vi "Xml_Load_Sequence.vi"(7 "Version String":string, 8 "error in (no error)":errorcluster, 10 "XML Path":path=path "D:/TEST.xml", 11 "Refnum Clust":refnum<vi>) -> (0 "error out":errorcluster)   [LabVIEW 2018]
uses:
  controls/SEQUENCE_Inputs.ctl
  controls/EXCIT_Inputs.ctl
  controls/DATA_Inputs.ctl
  controls/TIMING_Inputs.ctl
  controls/PROCESSING_Inputs.ctl
  controls/TRAPPING_Inputs.ctl
panel:
  in  "SEQUENCE Inputs":T1={"EXCIT Inputs"={"Number of Excitations"=1, "Script Text"="", "Table of Waveforms"=[]}, "DATA Inputs"={"Record Length"=524000, "Sample Rate"=2000000.0, "Data Type"=0, "Vertical Range"=10.0, "Acquisition Duration"=262.0}, "TIMING Inputs"={"Number of Acquisitions "=1, "Number of Accumulations"=1, "Table of Waveforms"=[], "Script Text"=""}, "PROCESSING Inputs"={"Reference Mass"=300.0939, "Cyclotron Freq"=255.727, "Magnetron Freq"=0.001}, "TRAPPING Inputs"={"Number of Channels"=4, "Init Values"=[2.0, 9.0, 2.0, 9.0], "Opening Values"=[0.0, 0.0, 0.0, 0.0], "Trapping Values"=[2.0, 9.0, 2.0, 9.0], "Emptying Values"=[-10.0, -10.0, -10.0, -10.0], "Adiabatic ON"=FALSE, "Adiabatic Duration"=100, "Adiabatic Waveforms"=["Adiabatic_None_2_2_2000", "Adiabatic_Ramp_9_0_2000", "Adiabatic_None_2_2_2000", "Adiabatic_RC_9_0_2000"], "Ions Refill ON"=FALSE, "Number of Ions Refills"=1, "Trapping Delay"=400.0, "Trapping Duration"=300.0}} {"TRAPPING Inputs"."Trapping Duration" min=2.0; "TRAPPING Inputs"."Trapping Delay" min=2.0; "TRAPPING Inputs"."Number of Ions Refills" min=1 max=1000; "TRAPPING Inputs"."Trapping Values" min=-10.0 max=10.0; "TRAPPING Inputs"."Init Values" min=-10.0 max=10.0; "TRAPPING Inputs"."Emptying Values" min=-10.0 max=10.0; "TRAPPING Inputs"."Opening Values" min=-10.0 max=10.0; "PROCESSING Inputs"."Magnetron Freq" format="%.5g"; "PROCESSING Inputs"."Cyclotron Freq" format="%.5g"; "PROCESSING Inputs"."Reference Mass" format="%.5g"; "TIMING Inputs"."Number of Accumulations" min=0 max=50 step=1; "TIMING Inputs"."Number of Acquisitions" min=1 max=10 step=1; "DATA Inputs"."Vertical Range" items=["0.2"=0.2, "0.4"=0.4, "1"=1.0, "2"=2.0, "4"=4.0, "10"=10.0]; "DATA Inputs"."Data Type" items=["I16", "DBL"]; "DATA Inputs"."Sample Rate" items=["1 MHz"=1000000.0, "2 MHz"=2000000.0, "5 MHz"=5000000.0, "10 MHz"=10000000.0, "20 MHz"=20000000.0, "25 MHz"=25000000.0, "50 MHz"=50000000.0, "100 MHz"=100000000.0]; "EXCIT Inputs"."Number of Excitations" min=1 max=10}
  # "GO_out"
  # "Gout"
  # "GI_in"
  # "Gin"
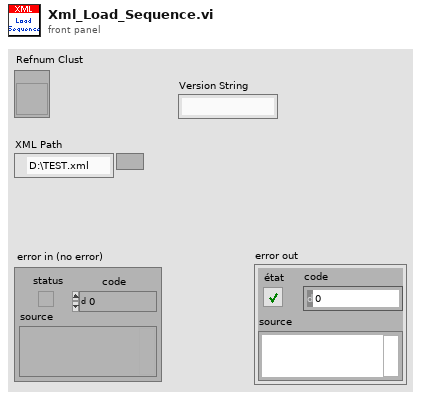
[diagram p1: front panel]
types:
  T1 = typedef "SEQUENCE_Inputs.ctl" = cluster{"EXCIT Inputs":T2, "DATA Inputs":T3, "TIMING Inputs":T4, "PROCESSING Inputs":T5, "TRAPPING Inputs":T6}
  T2 = typedef "EXCIT_Inputs.ctl" = cluster{"Number of Excitations":i32, "Script Text":string, "Table of Waveforms":string[]}
  T3 = typedef "DATA_Inputs.ctl" = cluster{"Record Length":i32, "Sample Rate":dbl, "Data Type":u8, "Vertical Range":dbl, "Acquisition Duration":dbl}
  T4 = typedef "TIMING_Inputs.ctl" = cluster{"Number of Acquisitions ":i16, "Number of Accumulations":i16, "Table of Waveforms":string[], "Script Text":string}
  T5 = typedef "PROCESSING_Inputs.ctl" = cluster{"Reference Mass":dbl, "Cyclotron Freq":dbl, "Magnetron Freq":dbl}
  T6 = typedef "TRAPPING_Inputs.ctl" = cluster{"Number of Channels":i32, "Init Values":dbl[], "Opening Values":dbl[], "Trapping Values":dbl[], "Emptying Values":dbl[], "Adiabatic ON":bool, "Adiabatic Duration":i32, "Adiabatic Waveforms":string[], "Ions Refill ON":bool, "Number of Ions Refills":i32, "Trapping Delay":dbl, "Trapping Duration":dbl}
  T7 = cluster{"Number of Channels":i32, "Init Values":dbl[], "Opening Values":dbl[], "Trapping Values":dbl[], "Emptying Values":dbl[], "Adiabatic ON":bool, "Adiabatic Duration":i32, "Adiabatic Waveforms":string[]}
  T8 = cluster{"Number Of Acquisitions ":i16, "Number Of Accumulations":i16, "Number Of Loops":i16, "Table of Waveforms":string[], "Script text":string}
  T9 = cluster{"Record Length":i32, "Sample Rate":dbl, "Type Of Data":u8, "Vertical Range":dbl, "Acquisition Duration":dbl}
  T10 = cluster{"Number of Excitations":i32, "Script text":string, "Table of Waveforms":string[]}
  T11 = cluster{"Reference Mass":dbl, "Cyclotron Freq":dbl, "Magnetron Freq":dbl}
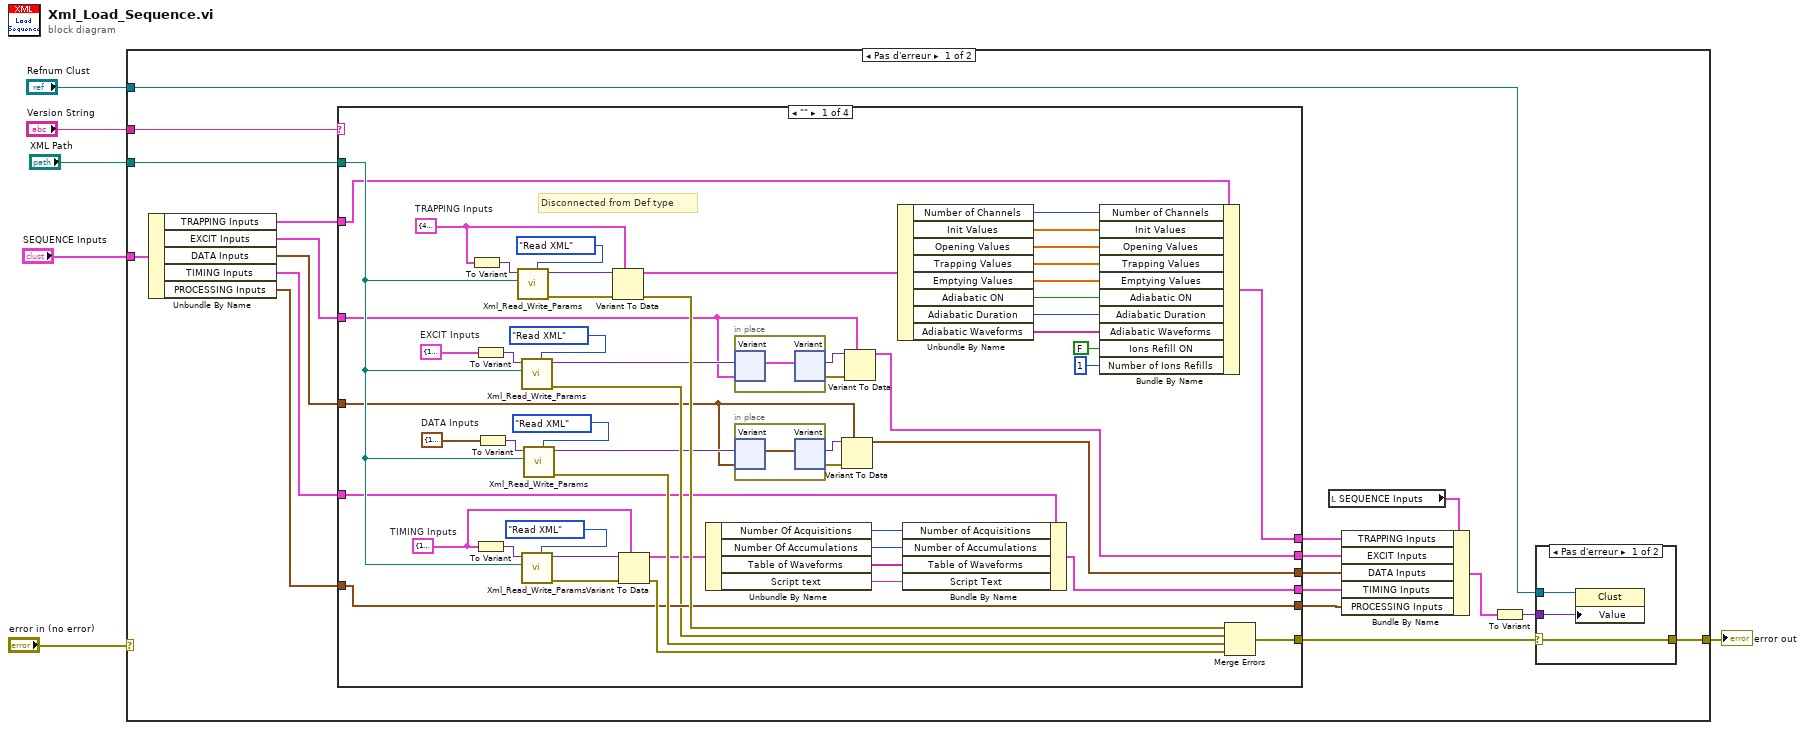
[diagram p0: block diagram]
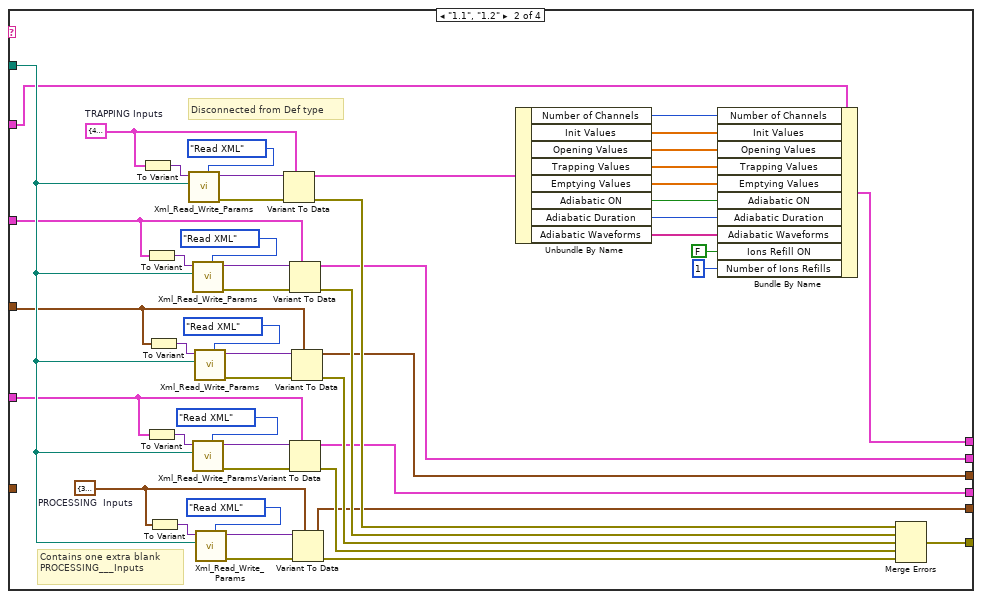
[diagram p2: hidden frame]
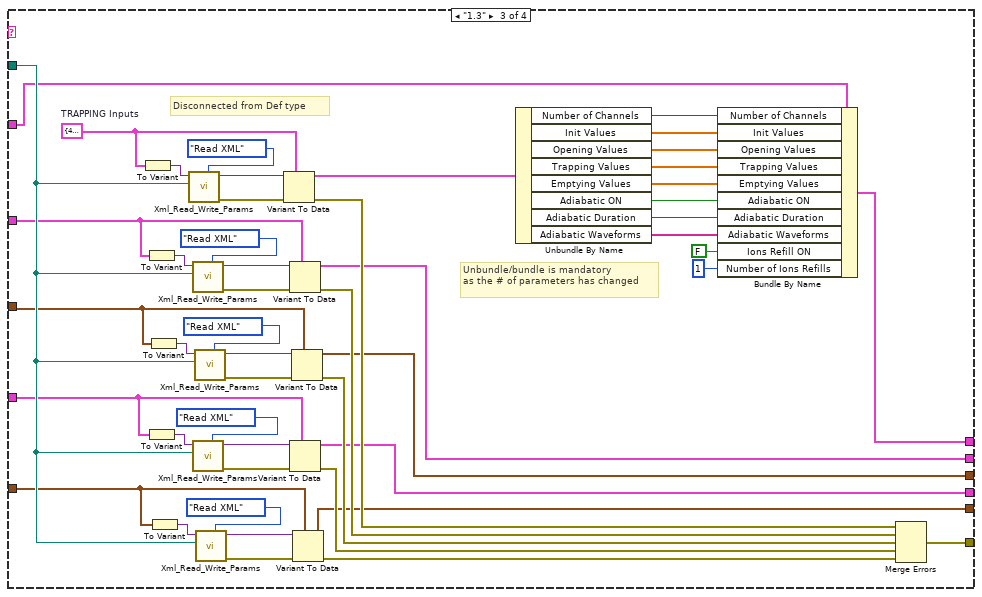
[diagram p3: hidden frame]
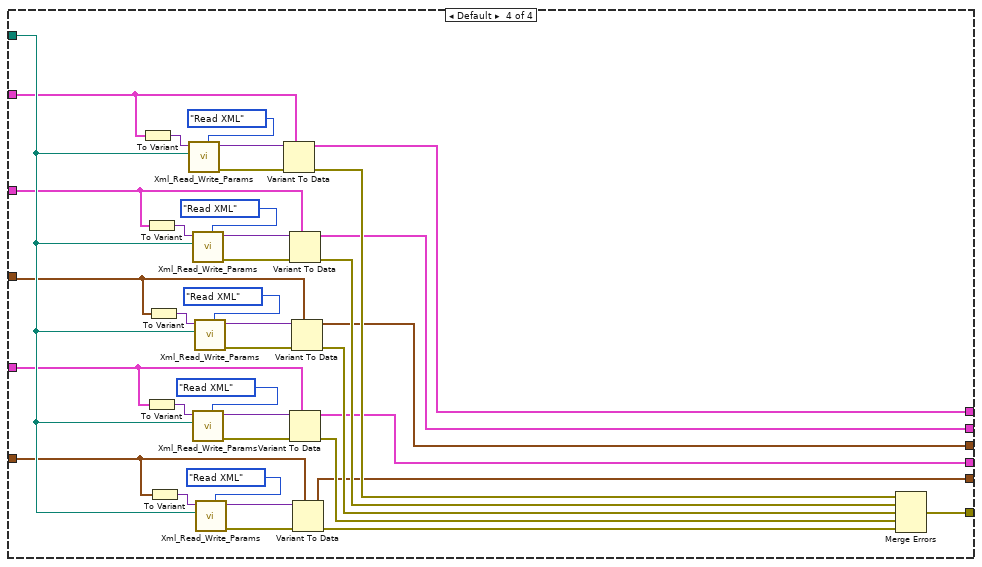
[diagram p4: hidden frame]
diagram:
  n1 = case shown="Pas d'erreur" "error in (no error)" {
    selector: "error in (no error)" -> [_ w220]
    tunnel: "XML Path" -> [w25 _]
    tunnel: [w22 w220] -> w4
    tunnel: "Version String" -> [w24 _]
    tunnel: "Refnum Clust" -> [w21 _]
    tunnel: "SEQUENCE Inputs" -> [w20 _]
    frame No Error {
      n2 = Unbundle By Name(w20) -> ("TRAPPING Inputs"=w19:T6, "EXCIT Inputs"=w18:T2, "DATA Inputs"=w17:T3, "TIMING Inputs"=w16:T4, "PROCESSING Inputs"=w15:T5)
      n3 = case shown="\"\"" w24 {
        tunnel: w25 -> [w62 w104 w153 w190]
        tunnel: [w78 w129 w178 w215] -> w23
        tunnel: w19 -> [w59 w92 w131 w188]
        tunnel: w18 -> [w52 w102 w151 w187]
        tunnel: w17 -> [w46 w101 w150 w186]
        tunnel: w16 -> [w39 w100 w149 w185]
        tunnel: w15 -> [w58 _ w148 w184]
        tunnel: [w60 w93 w133 w183] -> w14
        tunnel: [w37 w99 w147 w182] -> w9
        tunnel: [w47 w98 w146 w181] -> w8
        tunnel: [w38 w97 w145 w180] -> w13
        tunnel: [w58 w96 w144 w179] -> w12
        frame "" {
          w36 = T7 {"Number of Channels"=4, "Init Values"=[2.0, 9.0, 2.0, 9.0], "Opening Values"=[0.0, 0.0, 0.0, 0.0], "Trapping Values"=[2.0, 9.0, 2.0, 9.0], "Emptying Values"=[-10.0, -10.0, -10.0, -10.0], "Adiabatic ON"=FALSE, "Adiabatic Duration"=100, "Adiabatic Waveforms"=["Adiabatic_None_2_2_2000", "Adiabatic_Ramp_9_0_2000", "Adiabatic_None_2_2_2000", "Adiabatic_RC_9_0_2000"]}  # TRAPPING Inputs
          w45 = T8 {"Number Of Acquisitions "=1, "Number Of Accumulations"=1, "Number Of Loops"=1, "Table of Waveforms"=[], "Script text"=""}  # TIMING Inputs
          w51 = T9 {"Record Length"=100000, "Sample Rate"=10000000.0, "Type Of Data"=0, "Vertical Range"=10.0, "Acquisition Duration"=100000.0}  # DATA Inputs
          w57 = T10 {"Number of Excitations"=1, "Script text"="", "Table of Waveforms"=[]}  # EXCIT Inputs
          # "Disconnected from Def type"
          n4 = To Variant(anything=w36) -> (Variant=w77:variant)
          n5 = To Variant(anything=w57) -> (Variant=w72:variant)
          n6 = To Variant(anything=w45) -> (Variant=w65:variant)
          n7 = To Variant(anything=w51) -> (Variant=w71:variant)
          n8 = call "Xml_Read_Write_Params.vi"("Variant"=w77, "XML Path"=w62, "Command"=enum16{"Read XML", "Set", "Get", "Write XML"}."Read XML") -> ("Variant Output"=w75:variant, "error out"=w76:errorcluster)  [unwired: 4 in, 1 out]
          n9 = call "Xml_Read_Write_Params.vi"("Variant"=w72, "XML Path"=w62, "Command"=enum16{"Read XML", "Set", "Get", "Write XML"}."Read XML") -> ("Variant Output"=w55:variant, "error out"=w56:errorcluster)  [unwired: 4 in, 1 out]
          n10 = call "Xml_Read_Write_Params.vi"("Variant"=w65, "XML Path"=w62, "Command"=enum16{"Read XML", "Set", "Get", "Write XML"}."Read XML") -> ("Variant Output"=w67:variant, "error out"=w66:errorcluster)  [unwired: 4 in, 1 out]
          n11 = call "Xml_Read_Write_Params.vi"("Variant"=w71, "XML Path"=w62, "Command"=enum16{"Read XML", "Set", "Get", "Write XML"}."Read XML") -> ("Variant Output"=w50:variant, "error out"=w70:errorcluster)  [unwired: 4 in, 1 out]
          n12 = Variant To Data(error in=w76, type=w36, Variant=w75) -> (data=w35:T7, error out=w63:errorcluster)
          n13 = Variant To Data(error in=w66, type=w45, Variant=w67) -> (data=w40:T8, error out=w64:errorcluster)
          n14 = Unbundle By Name(w40) -> ("Number Of Acquisitions"=w44:i16, "Number Of Accumulations"=w43:i16, "Table of Waveforms"=w42:string[], "Script text"=w41:string)
          n15 = in-place "Structure Élément en place" {
            n16 = in-place-variant #1(w55, w52) -> (w80:T2)  [unwired: 1 out]
            n17 = in-place-variant #1(w80) -> (w53:variant, w54:errorcluster)
          }
          n18 = in-place "Structure Élément en place" {
            n19 = in-place-variant #2(w50, w46) -> (w79:T3)  [unwired: 1 out]
            n20 = in-place-variant #2(w79) -> (w48:variant, w49:errorcluster)
          }
          n21 = Variant To Data(error in=w49, type=w46, Variant=w48) -> (data=w47:T3)  [unwired: 1 out]
          n22 = Variant To Data(error in=w54, type=w52, Variant=w53) -> (data=w37:T2)  [unwired: 1 out]
          n23 = Unbundle By Name(w35) -> ("Number of Channels"=w34:i32, "Init Values"=w33:dbl[], "Opening Values"=w32:dbl[], "Trapping Values"=w31:dbl[], "Emptying Values"=w30:dbl[], "Adiabatic ON"=w29:bool, "Adiabatic Duration"=w28:i32, "Adiabatic Waveforms"=w27:string[])
          n24 = Bundle By Name(cluster=w39, "Number of Acquisitions"=w44, "Number of Accumulations"=w43, "Table of Waveforms"=w42, "Script Text"=w41) -> (w38:T4)
          n25 = Bundle By Name(cluster=w59, "Number of Channels"=w34, "Init Values"=w33, "Opening Values"=w32, "Trapping Values"=w31, "Emptying Values"=w30, "Adiabatic ON"=w29, "Adiabatic Duration"=w28, "Adiabatic Waveforms"=w27, "Ions Refill ON"=FALSE ("Ions Accumulation ON"), "Number of Ions Refills"=1) -> (w60:T6)
          n26 = Merge Errors(w63, w56, w70, w64) -> (w78:errorcluster)
        }
        frame "1.1", "1.2" {
          w90 = T7 {"Number of Channels"=4, "Init Values"=[2.0, 9.0, 2.0, 9.0], "Opening Values"=[0.0, 0.0, 0.0, 0.0], "Trapping Values"=[2.0, 9.0, 2.0, 9.0], "Emptying Values"=[-10.0, -10.0, -10.0, -10.0], "Adiabatic ON"=FALSE, "Adiabatic Duration"=100, "Adiabatic Waveforms"=["Adiabatic_None_2_2_2000", "Adiabatic_Ramp_9_0_2000", "Adiabatic_None_2_2_2000", "Adiabatic_RC_9_0_2000"]}  # TRAPPING Inputs
          w91 = T11 {"Reference Mass"=300.0939, "Cyclotron Freq"=255.727, "Magnetron Freq"=0.001}  # PROCESSING  Inputs
          # "Contains one extra blank\nPROCESSING___Inputs"
          # "Disconnected from Def type"
          n27 = To Variant(anything=w90) -> (Variant=w128:variant)
          n28 = To Variant(anything=w102) -> (Variant=w121:variant)
          n29 = To Variant(anything=w100) -> (Variant=w113:variant)
          n30 = To Variant(anything=w101) -> (Variant=w120:variant)
          n31 = To Variant(anything=w91) -> (Variant=w108:variant)
          n32 = call "Xml_Read_Write_Params.vi"("Variant"=w128, "XML Path"=w104, "Command"=enum16{"Read XML", "Set", "Get", "Write XML"}."Read XML") -> ("Variant Output"=w126:variant, "error out"=w127:errorcluster)  [unwired: 4 in, 1 out]
          n33 = call "Xml_Read_Write_Params.vi"("Variant"=w121, "XML Path"=w104, "Command"=enum16{"Read XML", "Set", "Get", "Write XML"}."Read XML") -> ("Variant Output"=w123:variant, "error out"=w122:errorcluster)  [unwired: 4 in, 1 out]
          n34 = call "Xml_Read_Write_Params.vi"("Variant"=w113, "XML Path"=w104, "Command"=enum16{"Read XML", "Set", "Get", "Write XML"}."Read XML") -> ("Variant Output"=w115:variant, "error out"=w114:errorcluster)  [unwired: 4 in, 1 out]
          n35 = call "Xml_Read_Write_Params.vi"("Variant"=w120, "XML Path"=w104, "Command"=enum16{"Read XML", "Set", "Get", "Write XML"}."Read XML") -> ("Variant Output"=w118:variant, "error out"=w119:errorcluster)  [unwired: 4 in, 1 out]
          n36 = call "Xml_Read_Write_Params.vi"("Variant"=w108, "XML Path"=w104, "Command"=enum16{"Read XML", "Set", "Get", "Write XML"}."Read XML") -> ("Variant Output"=w106:variant, "error out"=w107:errorcluster)  [unwired: 4 in, 1 out]
          n37 = Variant To Data(error in=w127, type=w90, Variant=w126) -> (data=w89:T7, error out=w109:errorcluster)
          n38 = Variant To Data(error in=w122, type=w102, Variant=w123) -> (data=w99:T2, error out=w110:errorcluster)
          n39 = Variant To Data(error in=w114, type=w100, Variant=w115) -> (data=w97:T4, error out=w112:errorcluster)
          n40 = Variant To Data(error in=w119, type=w101, Variant=w118) -> (data=w98:T3, error out=w111:errorcluster)
          n41 = Variant To Data(error in=w107, type=w91, Variant=w106) -> (data=w96:T11, error out=w103:errorcluster)
          n42 = Unbundle By Name(w89) -> ("Number of Channels"=w88:i32, "Init Values"=w87:dbl[], "Opening Values"=w86:dbl[], "Trapping Values"=w85:dbl[], "Emptying Values"=w84:dbl[], "Adiabatic ON"=w83:bool, "Adiabatic Duration"=w82:i32, "Adiabatic Waveforms"=w81:string[])
          n43 = Bundle By Name(cluster=w92, "Number of Channels"=w88, "Init Values"=w87, "Opening Values"=w86, "Trapping Values"=w85, "Emptying Values"=w84, "Adiabatic ON"=w83, "Adiabatic Duration"=w82, "Adiabatic Waveforms"=w81, "Ions Refill ON"=FALSE ("Ions Accumulation ON"), "Number of Ions Refills"=1) -> (w93:T6)
          n44 = Merge Errors(w109, w110, w111, w112, w103) -> (w129:errorcluster)
        }
        frame "1.3" {
          w132 = T7 {"Number of Channels"=4, "Init Values"=[2.0, 9.0, 2.0, 9.0], "Opening Values"=[0.0, 0.0, 0.0, 0.0], "Trapping Values"=[2.0, 9.0, 2.0, 9.0], "Emptying Values"=[-10.0, -10.0, -10.0, -10.0], "Adiabatic ON"=FALSE, "Adiabatic Duration"=100, "Adiabatic Waveforms"=["Adiabatic_None_2_2_2000", "Adiabatic_Ramp_9_0_2000", "Adiabatic_None_2_2_2000", "Adiabatic_RC_9_0_2000"]}  # TRAPPING Inputs
          # "Disconnected from Def type"
          # "Unbundle/bundle is mandatory\nas the # of parameters has changed"
          n45 = To Variant(anything=w132) -> (Variant=w177:variant)
          n46 = To Variant(anything=w151) -> (Variant=w170:variant)
          n47 = To Variant(anything=w149) -> (Variant=w162:variant)
          n48 = To Variant(anything=w150) -> (Variant=w169:variant)
          n49 = To Variant(anything=w148) -> (Variant=w157:variant)
          n50 = call "Xml_Read_Write_Params.vi"("Variant"=w177, "XML Path"=w153, "Command"=enum16{"Read XML", "Set", "Get", "Write XML"}."Read XML") -> ("Variant Output"=w175:variant, "error out"=w176:errorcluster)  [unwired: 4 in, 1 out]
          n51 = call "Xml_Read_Write_Params.vi"("Variant"=w170, "XML Path"=w153, "Command"=enum16{"Read XML", "Set", "Get", "Write XML"}."Read XML") -> ("Variant Output"=w172:variant, "error out"=w171:errorcluster)  [unwired: 4 in, 1 out]
          n52 = call "Xml_Read_Write_Params.vi"("Variant"=w162, "XML Path"=w153, "Command"=enum16{"Read XML", "Set", "Get", "Write XML"}."Read XML") -> ("Variant Output"=w164:variant, "error out"=w163:errorcluster)  [unwired: 4 in, 1 out]
          n53 = call "Xml_Read_Write_Params.vi"("Variant"=w169, "XML Path"=w153, "Command"=enum16{"Read XML", "Set", "Get", "Write XML"}."Read XML") -> ("Variant Output"=w167:variant, "error out"=w168:errorcluster)  [unwired: 4 in, 1 out]
          n54 = call "Xml_Read_Write_Params.vi"("Variant"=w157, "XML Path"=w153, "Command"=enum16{"Read XML", "Set", "Get", "Write XML"}."Read XML") -> ("Variant Output"=w155:variant, "error out"=w156:errorcluster)  [unwired: 4 in, 1 out]
          n55 = Variant To Data(error in=w176, type=w132, Variant=w175) -> (data=w134:T7, error out=w158:errorcluster)
          n56 = Variant To Data(error in=w171, type=w151, Variant=w172) -> (data=w147:T2, error out=w159:errorcluster)
          n57 = Variant To Data(error in=w163, type=w149, Variant=w164) -> (data=w145:T4, error out=w161:errorcluster)
          n58 = Variant To Data(error in=w168, type=w150, Variant=w167) -> (data=w146:T3, error out=w160:errorcluster)
          n59 = Variant To Data(error in=w156, type=w148, Variant=w155) -> (data=w144:T5, error out=w152:errorcluster)
          n60 = Unbundle By Name(w134) -> ("Number of Channels"=w143:i32, "Init Values"=w142:dbl[], "Opening Values"=w141:dbl[], "Trapping Values"=w140:dbl[], "Emptying Values"=w139:dbl[], "Adiabatic ON"=w138:bool, "Adiabatic Duration"=w137:i32, "Adiabatic Waveforms"=w136:string[])
          n61 = Bundle By Name(cluster=w131, "Number of Channels"=w143, "Init Values"=w142, "Opening Values"=w141, "Trapping Values"=w140, "Emptying Values"=w139, "Adiabatic ON"=w138, "Adiabatic Duration"=w137, "Adiabatic Waveforms"=w136, "Ions Refill ON"=FALSE ("Ions Accumulation ON"), "Number of Ions Refills"=1) -> (w133:T6)
          n62 = Merge Errors(w158, w159, w160, w161, w152) -> (w178:errorcluster)
        }
        frame Default {
          n63 = To Variant(anything=w188) -> (Variant=w214:variant)
          n64 = To Variant(anything=w187) -> (Variant=w207:variant)
          n65 = To Variant(anything=w185) -> (Variant=w199:variant)
          n66 = To Variant(anything=w186) -> (Variant=w206:variant)
          n67 = To Variant(anything=w184) -> (Variant=w194:variant)
          n68 = call "Xml_Read_Write_Params.vi"("Variant"=w214, "XML Path"=w190, "Command"=enum16{"Read XML", "Set", "Get", "Write XML"}."Read XML") -> ("Variant Output"=w212:variant, "error out"=w213:errorcluster)  [unwired: 4 in, 1 out]
          n69 = call "Xml_Read_Write_Params.vi"("Variant"=w207, "XML Path"=w190, "Command"=enum16{"Read XML", "Set", "Get", "Write XML"}."Read XML") -> ("Variant Output"=w209:variant, "error out"=w208:errorcluster)  [unwired: 4 in, 1 out]
          n70 = call "Xml_Read_Write_Params.vi"("Variant"=w199, "XML Path"=w190, "Command"=enum16{"Read XML", "Set", "Get", "Write XML"}."Read XML") -> ("Variant Output"=w201:variant, "error out"=w200:errorcluster)  [unwired: 4 in, 1 out]
          n71 = call "Xml_Read_Write_Params.vi"("Variant"=w206, "XML Path"=w190, "Command"=enum16{"Read XML", "Set", "Get", "Write XML"}."Read XML") -> ("Variant Output"=w204:variant, "error out"=w205:errorcluster)  [unwired: 4 in, 1 out]
          n72 = call "Xml_Read_Write_Params.vi"("Variant"=w194, "XML Path"=w190, "Command"=enum16{"Read XML", "Set", "Get", "Write XML"}."Read XML") -> ("Variant Output"=w192:variant, "error out"=w193:errorcluster)  [unwired: 4 in, 1 out]
          n73 = Variant To Data(error in=w213, type=w188, Variant=w212) -> (data=w183:T6, error out=w195:errorcluster)
          n74 = Variant To Data(error in=w208, type=w187, Variant=w209) -> (data=w182:T2, error out=w196:errorcluster)
          n75 = Variant To Data(error in=w200, type=w185, Variant=w201) -> (data=w180:T4, error out=w198:errorcluster)
          n76 = Variant To Data(error in=w205, type=w186, Variant=w204) -> (data=w181:T3, error out=w197:errorcluster)
          n77 = Variant To Data(error in=w193, type=w184, Variant=w192) -> (data=w179:T5, error out=w189:errorcluster)
          n78 = Merge Errors(w195, w196, w197, w198, w189) -> (w215:errorcluster)
        }
      }
      n79 = local read "SEQUENCE Inputs"() -> (w7:T1)
      n80 = Bundle By Name(cluster=w7, "TRAPPING Inputs"=w14, "EXCIT Inputs"=w9, "DATA Inputs"=w8, "TIMING Inputs"=w13, "PROCESSING Inputs"=w12) -> (w11:T1)
      n81 = To Variant(anything=w11) -> (Variant=w10:variant)
      n82 = case shown="Pas d'erreur" w23 {
        selector: w23 -> [w217 w219]
        tunnel: w21 -> [w218 _]
        tunnel: [w217 w219] -> w22
        tunnel: w10 -> [w216 _]
        frame No Error {
          n83 = property class="Clust"(reference=w218, "Value"=w216) -> ()  [unwired: 1 in, 2 out]
        }
        frame Error {
        }
      }
    }
    frame Error {
    }
  }
  "error out" <- w4
